vi "One or More Tolerant Inputs.vi"(8 "error in (no error)":errorcluster, 10 "Tolerance":dbl, 11 "Mock in":refnum<class "Mock.lvclass">) -> (0 "error out":errorcluster, 3 "Mock out":refnum<class "Mock.lvclass">)   [LabVIEW 2020, in "One or More.lvclass"]
uses:
  Framework/Mock/Mock.lvclass
  Comparators/Identical Arguments Comparator/Identical Inputs Comparator.lvclass
  C:/git/astemes-lmock/source/Core/Comparator/Comparator.lvclass
  One or More.lvclass
  C:/git/astemes-lmock/source/Core/Expectation/Expectation.lvclass
  One or More.lvclass/One or More.ctl
  Comparators/Tolerant Numeric Argument Comparator/Tolerant Numeric Input Comparator.lvclass
  C:/git/astemes-lmock/source/Comparators/Tolerant Numeric Argument Comparator/Tolerant Numeric Input Comparator.lvclass
  C:/git/astemes-lmock/source/Expectations/One or More/One or More.lvclass
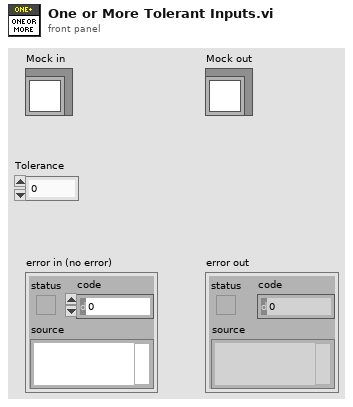
[diagram p1: front panel]
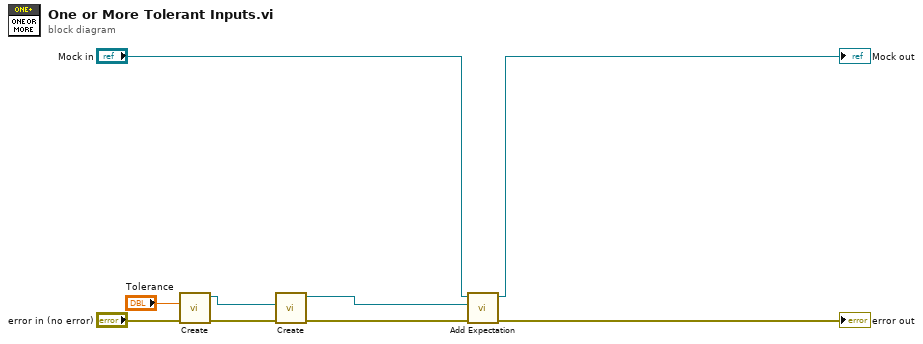
[diagram p0: block diagram]
diagram:
  n1 = call "Create.vi"("error in (no error)"="error in (no error)", "Tolerance"="Tolerance") -> ("error out"=w3:errorcluster, "Tolerant Numeric Comparator Out"=w2:refnum<class "Tolerant Numeric Input Comparator.lvclass">)  [unwired: 8 in]
  n2 = call "Create.vi"("error in (no error)"=w3, "Comparator"=w2) -> ("error out"=w5:errorcluster, "One or More"=w4:refnum<class "One or More.lvclass">)  [unwired: 8 in]
  n3 = call-dynamic "Add Expectation.vi"("error in (no error)"=w5, "Expectations"=w4, "Mock in"="Mock in") -> ("error out"=→"error out":errorcluster, "Mock out"=→"Mock out":refnum<class "Mock.lvclass">)  [unwired: 7 in]
